vi "Read start time.vi"(8 "error in":errorcluster, 11 "timing source in":refnum<class "absolute usec timing source.lvclass">) -> (0 "error out":errorcluster, 2 "start time":timestamp, 3 "timing source out":refnum<class "absolute usec timing source.lvclass">)   [LabVIEW 2013, in "absolute usec timing source.lvclass"]
doc: "Returns the start time of an absolute timing source"
uses:
  absolute usec timing source.lvclass
  absolute usec timing source.lvclass/absolute usec timing source.ctl
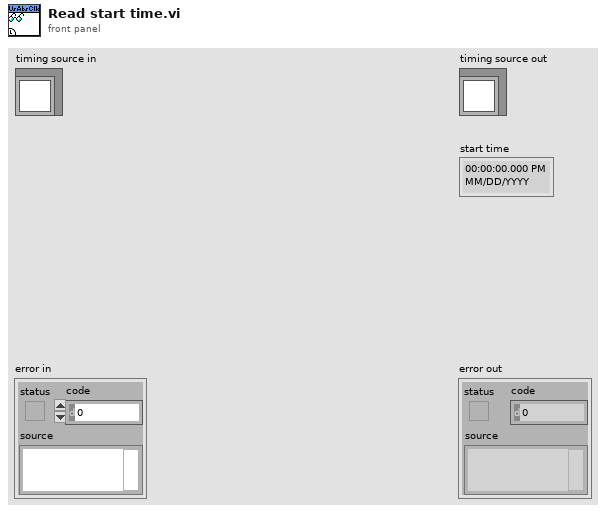
[diagram p1: front panel]
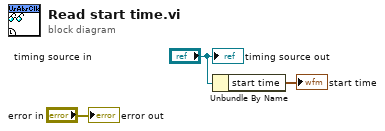
[diagram p0: block diagram]
diagram:
  n1 = Unbundle By Name("timing source in") -> ("start time"=→"start time":timestamp)
  "error out" <- "error in"
  "timing source out" <- "timing source in"
